vi "constants.vi"() -> ()   [LabVIEW 2012]
uses:
  typedefs/fg_typedef.ctl
panel:
  out "output":dbl
  in  "Constant Name":string
  in  "Menu":T1
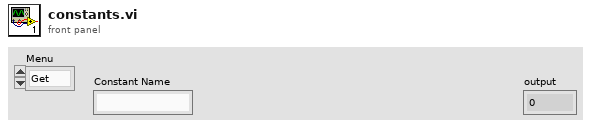
[diagram p1: front panel]
types:
  T1 = typedef "fg_typedef.ctl" = enum16{"Get", "Set"}
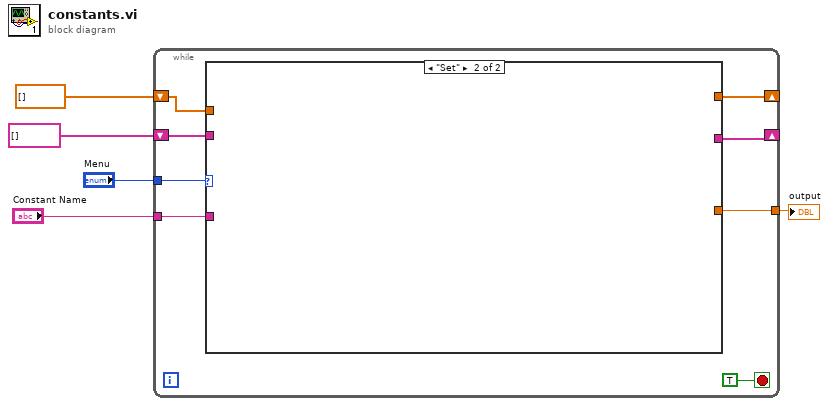
[diagram p0: block diagram]
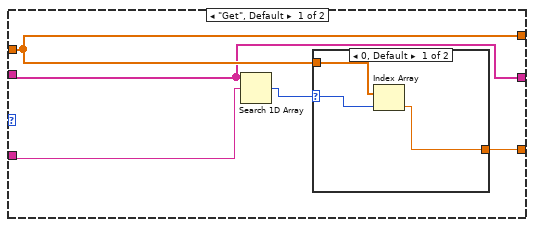
[diagram p2: hidden frame]
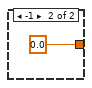
[diagram p3: hidden frame]
diagram:
  n1 = while {
    tunnel: "Menu" -> [w12]
    shift-right: [w8] -> _
    shift-left: dbl[] [] -> [w11]
    tunnel: "Constant Name" -> [w10]
    shift-right: [w7] -> _
    shift-left: string[] [] -> [w9]
    tunnel: [w6] -> w1
    stop <- TRUE stop-if-true
    n2 = case shown="\"Set\"" w12 {
      tunnel: w11 -> [w16 _]
      tunnel: w10 -> [w17 _]
      tunnel: w9 -> [w15 _]
      tunnel: [w16 _] -> w8
      tunnel: [w15 _] -> w7
      tunnel: [w14 _] -> w6
      frame "Get", Default {
        n3 = Search 1D Array(1D array=w15, element=w17) -> (index of element=w18:i32)  [unwired: 1 in]
        n4 = case shown="0, Default" w18 {
          selector: w18 -> [w20 _]
          tunnel: [w19 0.0] -> w14
          tunnel: w16 -> [w21 _]
          frame 0, Default {
            n5 = Index Array(array=w21, index=w20) -> (element=w19:dbl)
          }
          frame -1 {
          }
        }
      }
      frame "Set" {
      }
    }
  }
  "output" <- w1
